vi "Write Log Root.vi"(8 "error in (no error)":errorcluster, 10 "Log Root":path, 11 "File Logger in":refnum<class "File Logger.lvclass">) -> (0 "error out":errorcluster, 3 "File Logger out":refnum<class "File Logger.lvclass">)   [LabVIEW 2020, in "Logging.lvlib" / "File Logger.lvclass"]
uses:
  File Logger.lvclass
  File Logger.lvclass/File Logger.ctl
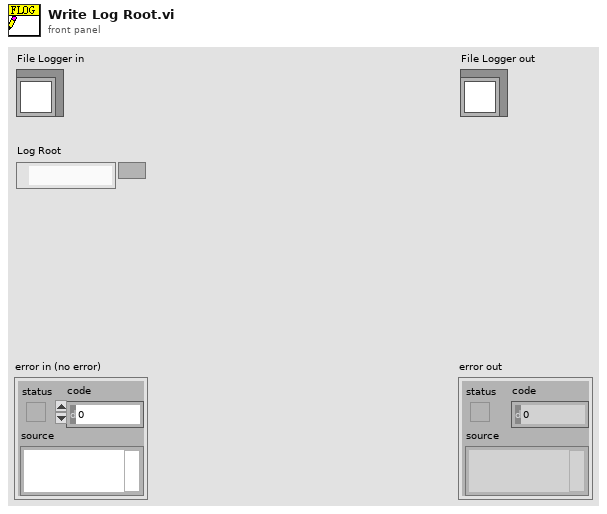
[diagram p1: front panel]
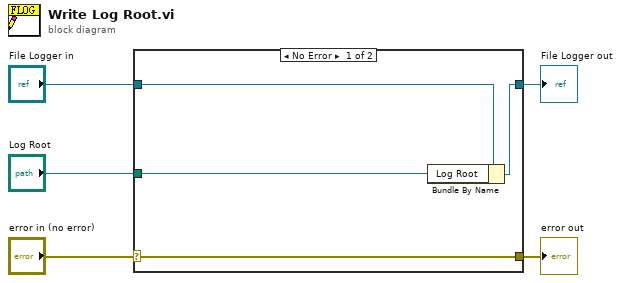
[diagram p0: block diagram]
diagram:
  n1 = case shown="No Error" "error in (no error)" {
    selector: "error in (no error)" -> [w9 w10]
    tunnel: [w9 w10] -> w4
    tunnel: [w7 w11] -> w2
    tunnel: "File Logger in" -> [w8 w11]
    tunnel: "Log Root" -> [w6 _]
    frame No Error {
      n2 = Bundle By Name(cluster=w8, "Log Root"=w6) -> (w7:refnum<class "File Logger.lvclass">)
    }
    frame Error {
    }
  }
  "error out" <- w4
  "File Logger out" <- w2
